vi "Bundle.vi"(8 "error in":errorcluster, 9 "Instrument String":string, 10 "Msg Name":string, 11 "Time Stamp":timestamp) -> (3 "Instrument Error Data out":refnum<class "Instrument Error Data.lvclass">)   [LabVIEW 2020, in "Instrument Handler.lvlib" / "Instrument Error Data.lvclass"]
doc: "Populate the Instrument Error Data."
uses:
  Instrument Error Data.lvclass
  Instrument Error Data.lvclass/Instrument Error Data.ctl
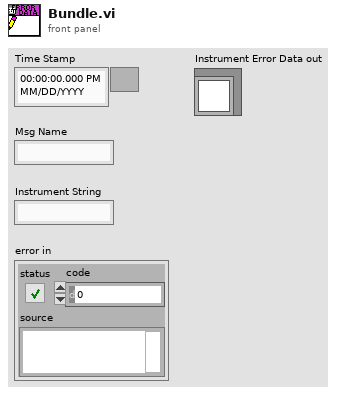
[diagram p1: front panel]
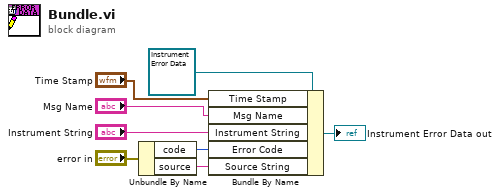
[diagram p0: block diagram]
diagram:
  n1 = Unbundle By Name("error in") -> ("code"=w2:i32, "source"=w1:string)
  n2 = Bundle By Name(cluster=refnum<class "Instrument Error Data.lvclass"> refnum ("Instrument Error Data out 2"), "Time Stamp"="Time Stamp", "Msg Name"="Msg Name", "Instrument String"="Instrument String", "Error Code"=w2, "Source String"=w1) -> (→"Instrument Error Data out":refnum<class "Instrument Error Data.lvclass">)
